vi "Import from JSON RTM.vi"(8 "error in":errorcluster, 11 "Node Ptr":u64 format="%.0x") -> (0 "error out":errorcluster)   [LabVIEW 2026, in "NIDMM System Explorer.lvlib"]
uses:
  NIDMM System Explorer.lvlib
  <vilib>/NI/VeriStand Custom Device Serialization/System Explorer Action.ctl
  NationalInstruments.VeriStand.SystemDefinitionAPI
  <vilib>/NI/VeriStand Custom Device Serialization/Custom Device Serialization.lvlib
panel:
  in  "Tag":string
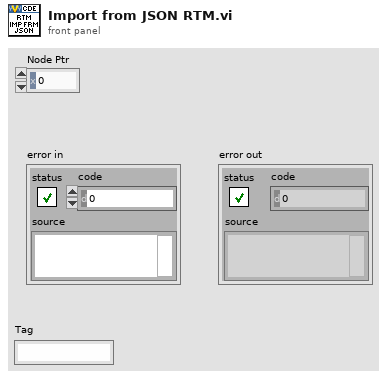
[diagram p1: front panel]
types:
  T1 = typedef "Custom Device Serialization.lvlib/System Explorer Action.ctl" = u16
  T2 = typedef "Custom Device API.lvlib/Custom Device Item Ref.ctl" = u64
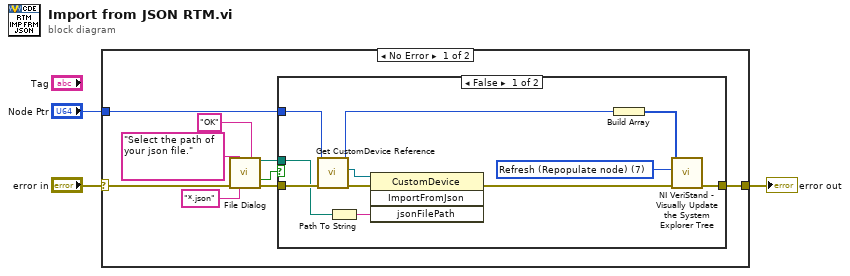
[diagram p0: block diagram]
diagram:
  n1 = case shown="No Error" "error in" {
    selector: "error in" -> [w12 w25]
    tunnel: [w11 w25] -> w1
    tunnel: "Node Ptr" -> [w10 _]
    frame No Error {
      n2 = call "File Dialog"("prompt"="Select the path of your json file.", "button label"="OK", "error in"=w12, "pattern (all files)"="*.json") -> ("selected path"=w7:path, "cancelled"=w4:bool, "error out"=w6:errorcluster)  [unwired: 8 in, 1 out]
      n3 = case shown="False" w4 {
        tunnel: w7 -> [w22 _]
        tunnel: w6 -> [w23 w24]
        tunnel: [w14 w24] -> w11
        tunnel: w10 -> [w21 _]
        frame False {
          w16 = T1 7 items=["Refresh (Add)"=5, "Refresh (Repopulate node)"=7] ("Action")
          n4 = call "Get CustomDevice Reference.vi"("error in"=w23, "Node Ptr"=w21) -> ("error out"=w19:errorcluster, "Custom Device"=w18:refnum<k24>, "Node Ptr"=w13:T2)  [unwired: 7 in]
          n5 = Path To String(path=w22) -> (string=w20:string)
          n6 = invoke class="CustomDevice" method="ImportFromJson"(reference=w18, error in=w19, "jsonFilePath"=w20) -> (error out=w15:errorcluster)  [unwired: 1 in, 3 out]
          n7 = Build Array(w13) -> (w17:T2[])
          n8 = call <vilib>:"NI VeriStand - Visually Update the System Explorer Tree.vi"("error in (no error)"=w15, "Action"=w16, "Node IDs"=w17) -> ("error out"=w14:errorcluster)  [unwired: 8 in]
        }
        frame True {
        }
      }
    }
    frame Error {
    }
  }
  "error out" <- w1
